vi "GenerateLogfilepath.vi"(2 "Number":u32, 3 "Instrument":string="Sensors_DAQ1") -> (0 "Logfile Path DAQmx":path=path "C:/Labview Test Data/2018-08-08/Sensors_DAQ1_Log.tdms", 1 "Logfile Path":path=path "C:/Labview Test Data/2018-08-08/Sensors_DAQ1_Log.tdms")   [LabVIEW 2018]
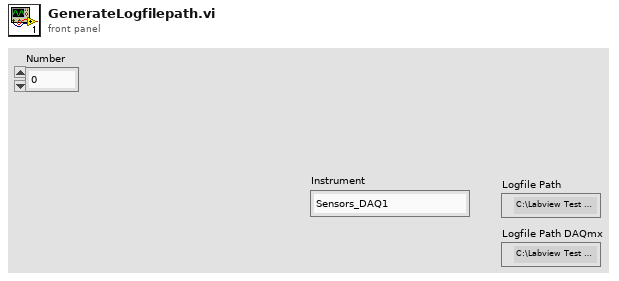
[diagram p1: front panel]
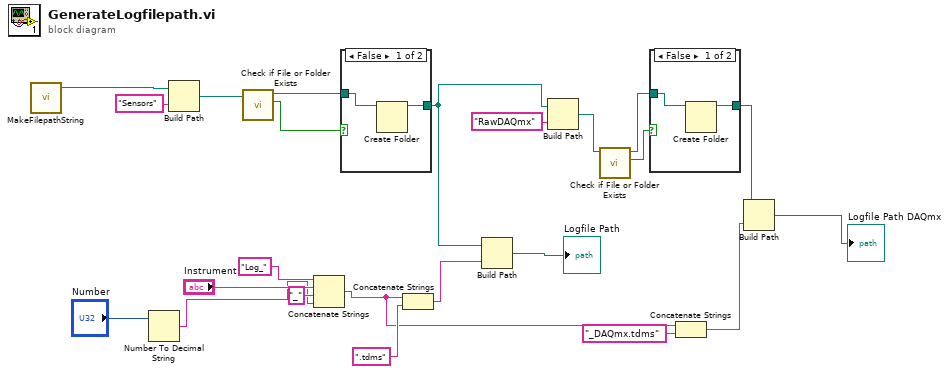
[diagram p0: block diagram]
diagram:
  n1 = call "MakeFilepathString.vi"() -> ("Date Folder"=w17:path)  [unwired: 6 in, 1 out]
  n2 = Number To Decimal String(number="Number") -> (decimal integer string=w18:string)  [unwired: 1 in]
  n3 = Build Path(base path=w17, name or relative path="Sensors") -> (appended path=w14:path)
  n4 = call <vilib>:"Check if File or Folder Exists.vi"("path"=w14) -> ("file or folder exists?"=w13:bool, "dup path"=w15:path)  [unwired: 8 in, 1 out]
  n5 = Concatenate Strings("Log_" ("string"), "Instrument", "_" ("string"), w18) -> (w4:string)
  n6 = case shown="False" w13 {
    tunnel: w15 -> [w25 w26]
    tunnel: [w24 w26] -> w11
    frame False {
      n7 = Create Folder(path (use dialog)=w25) -> (created path=w24:path)  [unwired: 2 in, 2 out]
    }
    frame True {
    }
  }
  n8 = Concatenate Strings(w4, ".tdms" ("string")) -> (w5:string)
  n9 = Build Path(base path=w11, name or relative path=w5) -> (appended path=→"Logfile Path":path)
  n10 = Build Path(base path=w11, name or relative path="RawDAQmx") -> (appended path=w10:path)
  n11 = call <vilib>:"Check if File or Folder Exists.vi"("path"=w10) -> ("file or folder exists?"=w8:bool, "dup path"=w9:path)  [unwired: 8 in, 1 out]
  n12 = case shown="False" w8 {
    tunnel: w9 -> [w28 w29]
    tunnel: [w27 w29] -> w7
    frame False {
      n13 = Create Folder(path (use dialog)=w28) -> (created path=w27:path)  [unwired: 2 in, 2 out]
    }
    frame True {
    }
  }
  n14 = Concatenate Strings(w4, "_DAQmx.tdms" ("string")) -> (w2:string)
  n15 = Build Path(base path=w7, name or relative path=w2) -> (appended path=→"Logfile Path DAQmx":path)
